vi "init.vi"(7 "Timeout Value (ms)":u32=2000, 8 "error in (no error)":errorcluster, 9 "ID query?":bool, 10 "Load default parameters?":bool, 11 "VISA resource name":refnum<visa-resource-name>) -> (0 "error out":errorcluster, 2 "ID string":string, 3 "VISA resource name out":refnum<visa-resource-name>)   [LabVIEW 2018, in "Inficon IC6.lvlib"]
doc: "Start the active process or continue a process that is in the STOP state."
uses:
  <instrlib>/Inficon IC6/Inficon IC6.lvlib
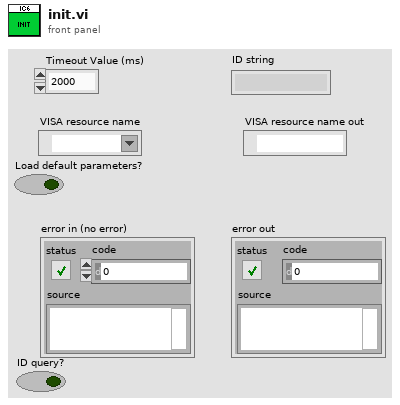
[diagram p1: front panel]
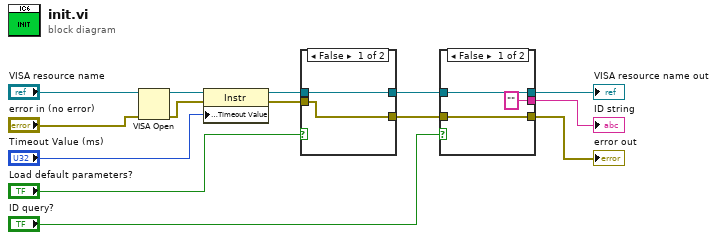
[diagram p0: block diagram]
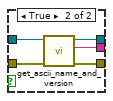
[diagram p2: hidden frame]
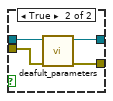
[diagram p3: hidden frame]
diagram:
  n1 = VISA Open(error in (no error)="error in (no error)", VISA resource name="VISA resource name") -> (VISA resource name=w11:refnum<visa-resource-name>, error out=w10:errorcluster)  [unwired: 3 in]
  n2 = property class="Instr"(reference=w11, error in=w10, "General Settings:Timeout Value"="Timeout Value (ms)") -> (reference out=w9:refnum<visa-resource-name>, error out=w8:errorcluster)
  n3 = case shown="False" "Load default parameters?" {
    tunnel: w9 -> [w15 w20]
    tunnel: w8 -> [w16 w19]
    tunnel: [w15 w18] -> w6
    tunnel: [w16 w17] -> w4
    frame False {
    }
    frame True {
      n4 = call <instrlib>:"deafult_parameters.vi"("error in (no error)"=w19, "VISA resource name"=w20) -> ("error out"=w17:errorcluster, "VISA resource name out"=w18:refnum<visa-resource-name>)  [unwired: 8 in]
    }
  }
  n5 = case shown="False" "ID query?" {
    tunnel: w6 -> [w23 w28]
    tunnel: w4 -> [w22 w27]
    tunnel: [w23 w26] -> w3
    tunnel: [w22 w25] -> w2
    tunnel: ["" ("ASCII name and version") w24] -> w1
    frame False {
    }
    frame True {
      n6 = call <instrlib>:"get_ascii_name_and_version.vi"("error in (no error)"=w27, "VISA resource name"=w28) -> ("error out"=w25:errorcluster, "ASCII name and version"=w24:string, "VISA resource name out"=w26:refnum<visa-resource-name>)  [unwired: 7 in]
    }
  }
  "error out" <- w2
  "VISA resource name out" <- w3
  "ID string" <- w1
